vi "Clear Scalar-Mixer Calibration Data.vi"(7 "Channel (1)":i32=1, 8 "error in (no error)":errorcluster, 10 "Clear (0: Calibration Coefficients)":u16(ring) items=["Calibration Coefficients", "Calibration Data"], 11 "VISA resource name":refnum<visa-resource-name>) -> (0 "error out":errorcluster, 3 "VISA resource name out":refnum<visa-resource-name>)   [LabVIEW 2018, in "Agilent ENA Series.lvlib"]
doc: "Clears the error coefficient or the measurement value of the Mechanical Cal kit for calibration when the frequency offset mode is enabled for selected channel. This command also clears the measurement value of the power meter.\n\nTo toggle the frequency offset mode, use agena Configure Frequency Offset.vi.\n\nNotes:\n(1) Settings that have been temporarily changed due to measurement for each standard (number of traces, measurement parameter, and so on) return to their original values.\n(2) This function does not clear the error coefficient when the frequency offset mode is disabled.\n(3) <b> This VI is not supported by the E5063A model.</b>"
uses:
  Agilent ENA Series.lvlib
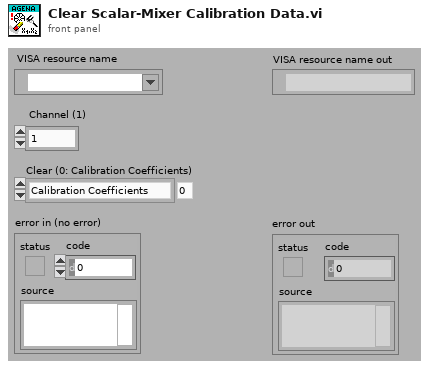
[diagram p1: front panel]
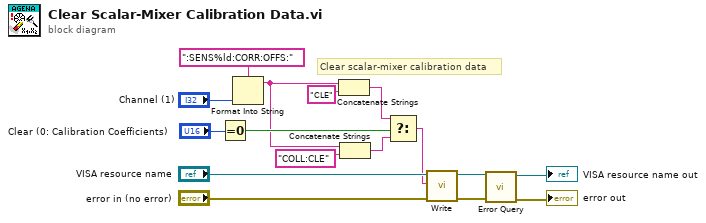
[diagram p0: block diagram]
diagram:
  # "Clear scalar-mixer calibration data"
  n1 = Equal To 0?(x="Clear (0: Calibration Coefficients)") -> (x = 0?=w11:bool)
  n2 = Format Into String(format string=":SENS%ld:CORR:OFFS:", "Channel (1)") -> (resulting string=w6:string)  [unwired: 2 in, 1 out]
  n3 = Concatenate Strings(w6, "CLE" ("string")) -> (w7:string)
  n4 = Concatenate Strings(w6, "COLL:CLE" ("string")) -> (w10:string)
  n5 = Select(t=w7, s=w11, f=w10) -> (s? t:f=w8:string)
  n6 = call "Write.vi"("error in (no error)"="error in (no error)", "String ()"=w8, "VISA resource name"="VISA resource name") -> ("error out"=w3:errorcluster, "VISA resource name out"=w4:refnum<visa-resource-name>)  [unwired: 6 in, 1 out]
  n7 = call "Error Query.vi"("error in (no error)"=w3, "VISA resource name"=w4) -> ("error out"=→"error out":errorcluster, "VISA resource name out"=→"VISA resource name out":refnum<visa-resource-name>)  [unwired: 6 in, 2 out]
